vi "Parse GLL Sentence.vi"(7 "date override":timestamp format="%<%x>T", 8 "error in (no error)":errorcluster, 11 "GLL sentence":string) -> (0 "error out":errorcluster, 3 "GLL data":T1 {"type of fix"."mode" items=["", "Simulator", "Not Valid", "Estimated", "Differential", "Autonomous"]; "status"."value" items=["Void", "Active"]; "time of fix"."time" format="%^<%.3X\n%x>T"})   [LabVIEW 2009]
doc: "Returns data contained in an NMEA sentence. You must manually select the polymorphic instance to use."
uses:
  typedefs/GLL Data.ctl
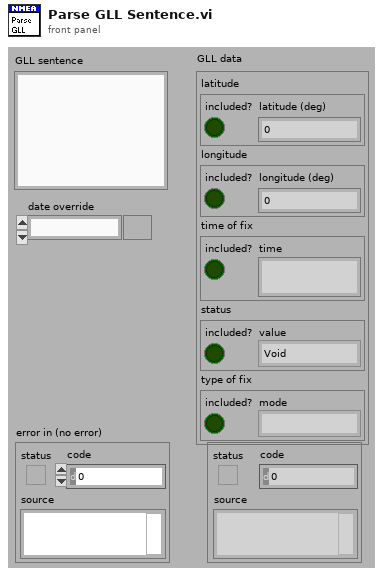
[diagram p1: front panel]
types:
  T1 = typedef "GLL Data.ctl" = cluster{"latitude":cluster{"included?":bool, "latitude (deg)":dbl}, "longitude":cluster{"included?":bool, "longitude (deg)":dbl}, "time of fix":cluster{"included?":bool, "time":timestamp}, "status":cluster{"included?":bool, "value":u16}, "type of fix":cluster{"included?":bool, "mode":u16}}
  T2 = typedef "LVDateTimeRec.ctl" = cluster{"fractional second":dbl, "second":i32, "minute":i32, "hour":i32, "day of month":i32, "month":i32, "year":i32, "day of week":i32, "day of year":i32, "DST":i32}
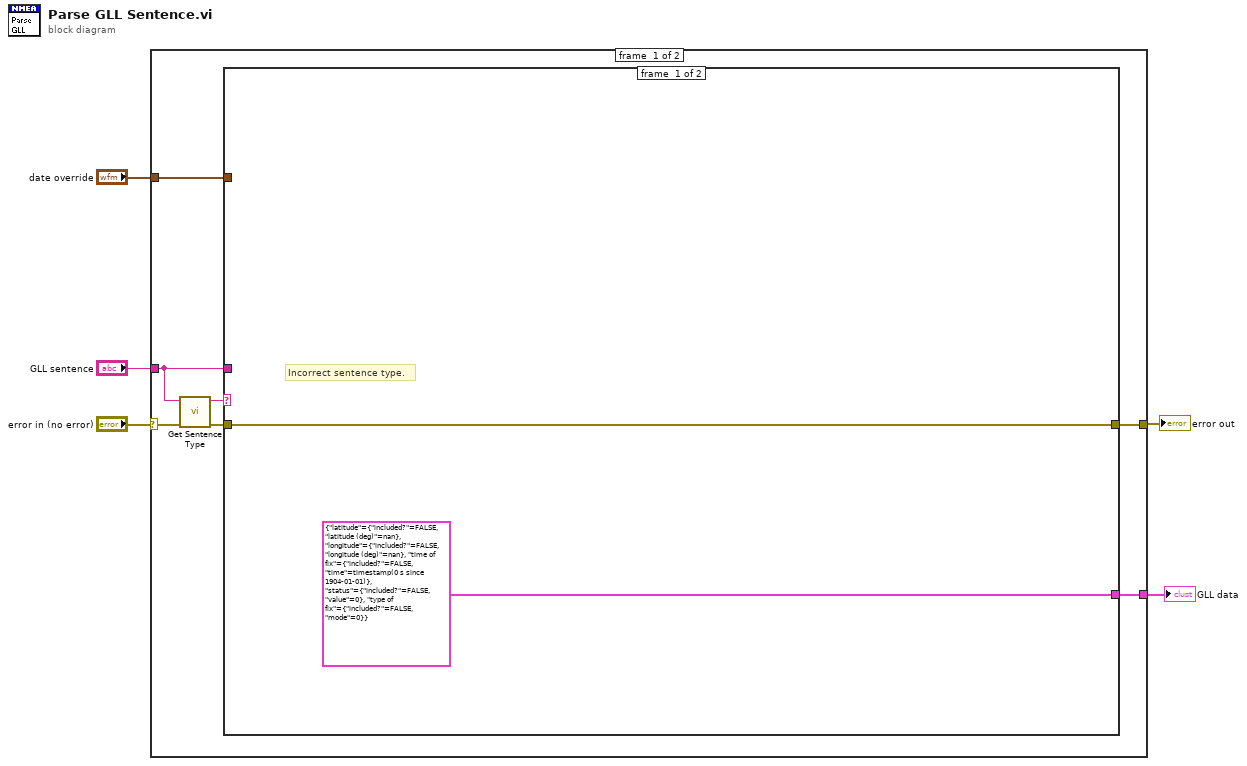
[diagram p0: block diagram]
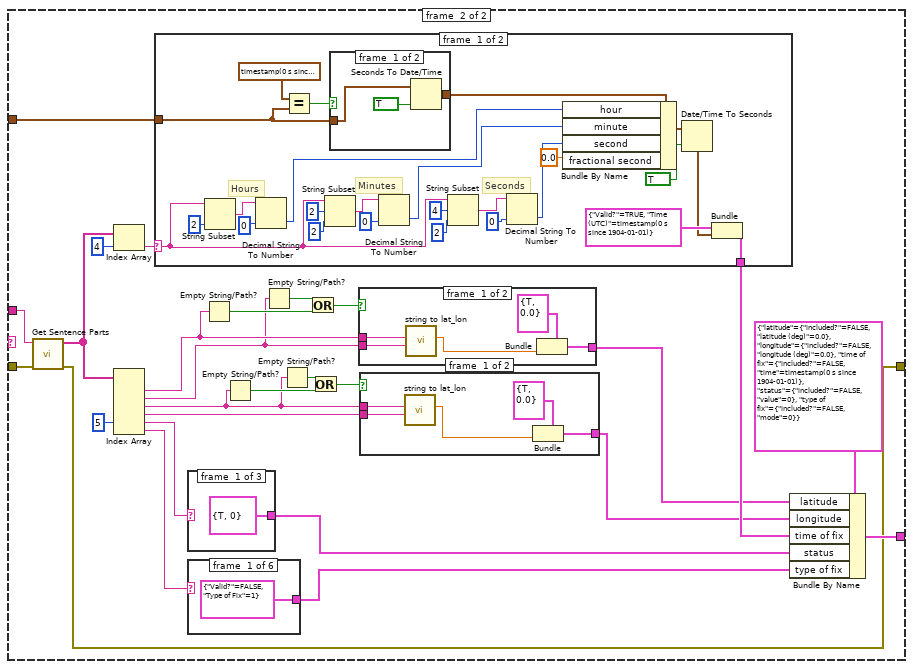
[diagram p2: hidden frame]
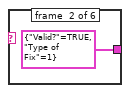
[diagram p3: hidden frame]
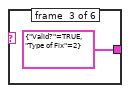
[diagram p4: hidden frame]
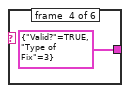
[diagram p5: hidden frame]
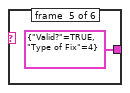
[diagram p6: hidden frame]
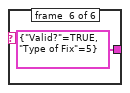
[diagram p7: hidden frame]
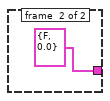
[diagram p8: hidden frame]
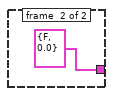
[diagram p9: hidden frame]
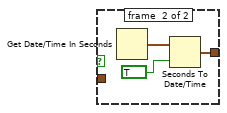
[diagram p10: hidden frame]
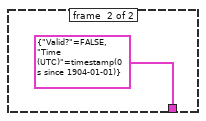
[diagram p11: hidden frame]
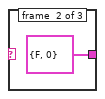
[diagram p12: hidden frame]
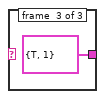
[diagram p13: hidden frame]
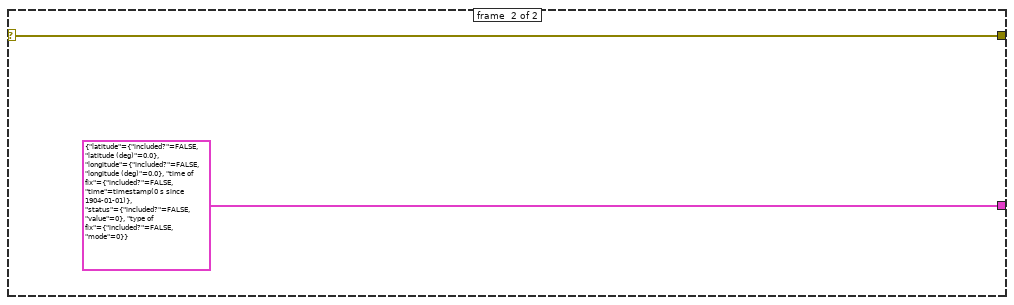
[diagram p14: hidden frame]
diagram:
  n1 = case shown="No Error" "error in (no error)" {
    selector: "error in (no error)" -> [w9 w96]
    tunnel: [w10 w96] -> w4
    tunnel: [w12 T1 {"latitude"={"included?"=FALSE, "latitude (deg)"=0.0}, "longitude"={"included?"=FALSE, "longitude (deg)"=0.0}, "time of fix"={"included?"=FALSE, "time"=timestamp(0 s since 1904-01-01)}, "status"={"included?"=FALSE, "value"=0}, "type of fix"={"included?"=FALSE, "mode"=0}} ("GLL Data")] -> w3
    tunnel: "GLL sentence" -> [w7 _]
    tunnel: "date override" -> [w11 _]
    frame #0 {
      n2 = call "Get Sentence Type.vi"("error in (no error)"=w9, "sentence"=w7) -> ("error out"=w8:errorcluster, "sentence type"=w6:string)  [unwired: 1 in, 7 out]
      n3 = case shown="\"GPGLL\"" w6 {
        tunnel: w7 -> [_ w17]
        tunnel: [T1 {"latitude"={"included?"=FALSE, "latitude (deg)"=nan}, "longitude"={"included?"=FALSE, "longitude (deg)"=nan}, "time of fix"={"included?"=FALSE, "time"=timestamp(0 s since 1904-01-01)}, "status"={"included?"=FALSE, "value"=0}, "type of fix"={"included?"=FALSE, "mode"=0}} ("GLL Data") w40] -> w12
        tunnel: w8 -> [w13 w38]
        tunnel: w11 -> [_ w28]
        tunnel: [w13 w15] -> w10
        frame #0 {
          # "Incorrect sentence type."
        }
        frame #1 {
          n4 = call "Get Sentence Parts.vi"("error in (no error)"=w38, "sentence"=w17) -> ("error out"=w15:errorcluster, "sentence data"=w16:string[])  [unwired: 1 in, 7 out]
          n5 = Index Array(array=w16, index=4) -> (element=w29:string)
          n6 = Index Array(array=w16, index #5=5 ("index")) -> (element #1=w25:string, element #2=w24:string, element #3=w27:string, element #4=w26:string, element #5=w36:string, element #6=w19:string)  [unwired: 5 in]
          n7 = case shown="\"False\", Default" w29 {
            selector: w29 -> [w64 _]
            tunnel: w28 -> [w82 _]
            tunnel: [w67 cluster{"Valid?":bool, "Time (UTC)":timestamp} {"Valid?"=FALSE, "Time (UTC)"=timestamp(0 s since 1904-01-01)} ("Time of Fix")] -> w23
            frame #0 {
              # "Seconds"
              # "Minutes"
              # "Hours"
              n8 = String Subset(string=w64, length (rest)=2 ("length (rest)")) -> (substring=w74:string)  [unwired: 1 out]
              n9 = Decimal String To Number(string=w74, default (0L)=0 ("default (0 DBL)")) -> (number=w68:i32)  [unwired: 2 out]
              n10 = Equal?(x=timestamp(0 s since 1904-01-01), y=w82) -> (x = y?=w84:bool)
              n11 = String Subset(string=w64, offset (0)=2, length (rest)=2 ("length (rest)")) -> (substring=w75:string)
              n12 = case shown="True" w84 {
                tunnel: w82 -> [w87 _]
                tunnel: [w86 w89] -> w72
                frame #0 {
                  n13 = Seconds To Date/Time(time stamp (now)=w87, to UTC (F)=TRUE) -> (date time rec=w86:T2)
                }
                frame #1 {
                  n14 = Get Date/Time In Seconds() -> (seconds since 1Jan1904=w90:timestamp)
                  n15 = Seconds To Date/Time(time stamp (now)=w90, to UTC (F)=TRUE) -> (date time rec=w89:T2)
                }
              }
              n16 = Decimal String To Number(string=w75, default (0L)=0 ("default (0 DBL)")) -> (number=w69:i32)  [unwired: 2 out]
              n17 = String Subset(string=w64, offset (0)=4, length (rest)=2 ("length (rest)")) -> (substring=w78:string)
              n18 = Decimal String To Number(string=w78, default (0L)=0 ("default (0 DBL)")) -> (number=w70:i32)  [unwired: 2 out]
              n19 = Bundle By Name(cluster=w72, "hour"=w68, "minute"=w69, "second"=w70, "fractional second"=0.0) -> (w71:T2)
              n20 = Date/Time To Seconds(1:TRUE, 2:w71) -> (0:w65:timestamp)
              n21 = Bundle(cluster=cluster{"Valid?":bool, "Time (UTC)":timestamp} {"Valid?"=TRUE, "Time (UTC)"=timestamp(0 s since 1904-01-01)} ("Time of Fix"), "Time (UTC)"=w65) -> (w67:cluster{"Valid?":bool, "Time (UTC)":timestamp})  [unwired: 1 out]
            }
            frame #1 {
            }
          }
          n22 = case shown="\"\", \" \", Default" w36 {
            tunnel: [cluster{"Valid?":bool, "Status":u16} {"Valid?"=TRUE, "Status"=0} ("Status") cluster{"Valid?":bool, "Status":u16} {"Valid?"=FALSE, "Status"=0} ("Status") cluster{"Valid?":bool, "Status":u16} {"Valid?"=TRUE, "Status"=1} ("Status")] -> w20
            frame #0 {
            }
            frame #1 {
            }
            frame #2 {
            }
          }
          n23 = case shown="\"\", \" \", Default" w19 {
            tunnel: [cluster{"Valid?":bool, "Type of Fix":u16} {"Valid?"=FALSE, "Type of Fix"=1} ("Type of Fix") cluster{"Valid?":bool, "Type of Fix":u16} {"Valid?"=TRUE, "Type of Fix"=1} ("Type of Fix") cluster{"Valid?":bool, "Type of Fix":u16} {"Valid?"=TRUE, "Type of Fix"=2} ("Type of Fix") cluster{"Valid?":bool, "Type of Fix":u16} {"Valid?"=TRUE, "Type of Fix"=3} ("Type of Fix") cluster{"Valid?":bool, "Type of Fix":u16} {"Valid?"=TRUE, "Type of Fix"=4} ("Type of Fix") cluster{"Valid?":bool, "Type of Fix":u16} {"Valid?"=TRUE, "Type of Fix"=5} ("Type of Fix")] -> w18
            frame #0 {
            }
            frame #1 {
            }
            frame #2 {
            }
            frame #3 {
            }
            frame #4 {
            }
            frame #5 {
            }
          }
          n24 = Empty String/Path?(string/path=w25) -> (empty?=w33:bool)
          n25 = Empty String/Path?(string/path=w27) -> (empty?=w32:bool)
          n26 = Empty String/Path?(string/path=w24) -> (empty?=w34:bool)
          n27 = Empty String/Path?(string/path=w27) -> (empty?=w31:bool)
          n28 = Or(x=w34, y=w33) -> (x .or. y?=w35:bool)
          n29 = Or(x=w31, y=w32) -> (x .or. y?=w30:bool)
          n30 = case shown="False" w35 {
            tunnel: [w56 cluster{"Valid?":bool, "Latitude (Deg)":dbl} {"Valid?"=FALSE, "Latitude (Deg)"=0.0} ("Latitude")] -> w22
            tunnel: w25 -> [w58 _]
            tunnel: w24 -> [w57 _]
            frame #0 {
              n31 = call "string to lat_lon.vi"("direction string"=w57, "numeric string for lat/lon"=w58) -> ("composite value"=w54:dbl)  [unwired: 1 in, 8 out]
              n32 = Bundle(cluster=cluster{"Valid?":bool, "Latitude (Deg)":dbl} {"Valid?"=TRUE, "Latitude (Deg)"=0.0} ("Latitude"), "Latitude (Deg)"=w54) -> (w56:cluster{"Valid?":bool, "Latitude (Deg)":dbl})  [unwired: 1 out]
            }
            frame #1 {
            }
          }
          n33 = case shown="False" w30 {
            tunnel: w26 -> [w52 _]
            tunnel: w27 -> [w51 _]
            tunnel: [w48 cluster{"Valid?":bool, "Longitude (Deg)":dbl} {"Valid?"=FALSE, "Longitude (Deg)"=0.0} ("Longitude")] -> w21
            frame #0 {
              n34 = call "string to lat_lon.vi"("direction string"=w52, "numeric string for lat/lon"=w51) -> ("composite value"=w50:dbl)  [unwired: 1 in, 8 out]
              n35 = Bundle(cluster=cluster{"Valid?":bool, "Longitude (Deg)":dbl} {"Valid?"=TRUE, "Longitude (Deg)"=0.0} ("Longitude"), "Longitude (Deg)"=w50) -> (w48:cluster{"Valid?":bool, "Longitude (Deg)":dbl})  [unwired: 1 out]
            }
            frame #1 {
            }
          }
          n36 = Bundle By Name(cluster=T1 {"latitude"={"included?"=FALSE, "latitude (deg)"=0.0}, "longitude"={"included?"=FALSE, "longitude (deg)"=0.0}, "time of fix"={"included?"=FALSE, "time"=timestamp(0 s since 1904-01-01)}, "status"={"included?"=FALSE, "value"=0}, "type of fix"={"included?"=FALSE, "mode"=0}} ("GLL Data"), "latitude"=w22, "longitude"=w21, "time of fix"=w23, "status"=w20, "type of fix"=w18) -> (w40:T1)
        }
      }
    }
    frame #1 {
    }
  }
  "error out" <- w4
  "GLL data" <- w3
